vi "analoog naar digitaal lrefectiesensor (SubVI).vi"(11 "Array in":dbl[](array[numeric])) -> (3 "Array out":i32[](array[numeric]))   [LabVIEW 2019]
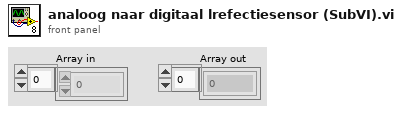
[diagram p1: front panel]
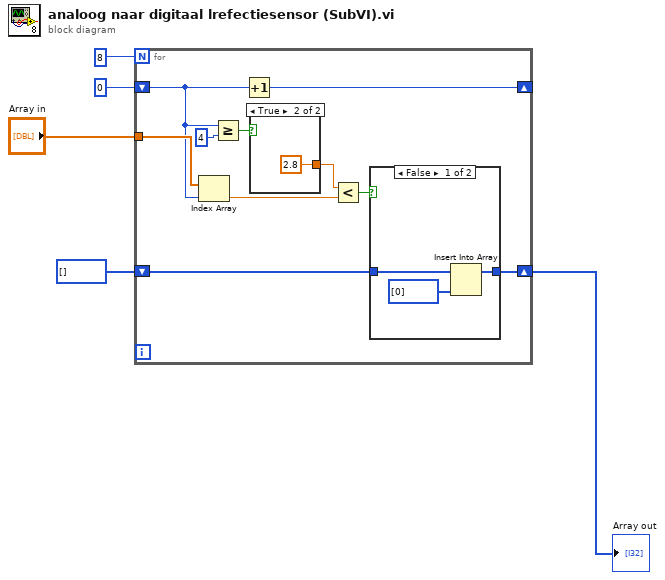
[diagram p0: block diagram]
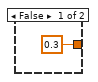
[diagram p2: hidden frame]
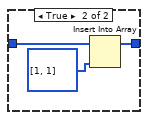
[diagram p3: hidden frame]
diagram:
  n1 = for {
    N: 8 -> [_]
    shift-right: [w14] -> w1
    shift-left: i32[] [] -> [w15]
    shift-right: [w12] -> _
    shift-left: 0 -> [w7]
    tunnel: "Array in" -> [w10]
    n2 = Index Array(array=w10, index=w7) -> (element=w11:dbl)
    n3 = Greater Or Equal?(x=w7, y=4) -> (x >= y?=w8:bool)
    n4 = Increment(x=w7) -> (x+1=w12:i32)
    n5 = case shown="True" w8 {
      tunnel: [0.3 2.8] -> w9
      frame False {
      }
      frame True {
      }
    }
    n6 = Less?(x=w9, y=w11) -> (x < y?=w13:bool)
    n7 = case shown="False" w13 {
      tunnel: w15 -> [w19 w21]
      tunnel: [w20 w23] -> w14
      frame False {
        n8 = Insert Into Array(array=w19, new element=i32[] [0]) -> (w20:i32[])  [unwired: 1 in]
      }
      frame True {
        n9 = Insert Into Array(array=w21, new element=i32[] [1, 1]) -> (w23:i32[])  [unwired: 1 in]
      }
    }
  }
  "Array out" <- w1
